vi "Accelerometer.vi"(1 "Mode":enum8{"Start", "Run", "Finish"}(ring)) -> (0 "Distances":cluster{"X":dbl, "Y":dbl, "Z":dbl})   [LabVIEW 2014]
uses:
  <vilib>/Rock Robotics/WPI/Accelerometer/InternalAccelerometer/WPI_AccelerometerInternalOpen.vi
  <vilib>/Analysis/NI_AALPro.lvlib
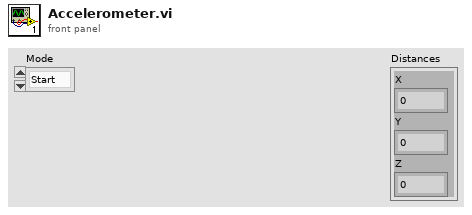
[diagram p1: front panel]
types:
  T1 = typedef "WPI_AccelerometerDevRef.ctl" = cluster{"DevStatus":errorcluster, "Controller":T2, "Scaling":T3, "Analog Channels":T4, "I2C Bus":T6, "SPI Bus":T7, "Accel Range":T8, "ADXL345 Axes":T9, "Handle":i32, "Device Address":u8, "Accel Type":enum16{"Analog", "ADXL345 I2C", "ADXL345 SPI", "Internal"}}
  T2 = typedef "FPGA_TypedefAnalogModule.ctl" = enum16{"Controller 1"}
  T3 = typedef "WPI_AccelerometerScaling.ctl" = cluster{"Gain (VoltsPerG)":dbl, "Center Voltage":dbl}
  T4 = typedef "WPI_AccelerometerAnalogChannels.ctl" = cluster{"X-Axis":T5, "Y-Axis":T5, "Z-Axis":T5}
  T5 = typedef "FPGA_AIChannel.ctl" = enum8{"AI 0", "AI 1", "AI 2", "AI 3", "AI MXP 0", "AI MXP 1", "AI MXP 2", "AI MXP 3", "Invalid"}
  T6 = typedef "i2c_bus.ctl" = enum16{"I2C On-Board", "I2C MXP", "Invalid"}
  T7 = typedef "spi_bus.ctl" = enum16{"SPI On-Board, CS0", "SPI On-Board, CS1", "SPI On-Board, CS2", "SPI On-Board, CS3", "SPI MXP", "Invalid"}
  T8 = typedef "ADXL345 Range.ctl" = u8
  T9 = typedef "WPI_AccelerometerADXL345 Axes.ctl" = cluster{"X-Axis":bool, "Y-Axis":bool, "Z-Axis":bool}
  T10 = cluster{"X-Axis":dbl, "Y-Axis":dbl, "Z-Axis":dbl}
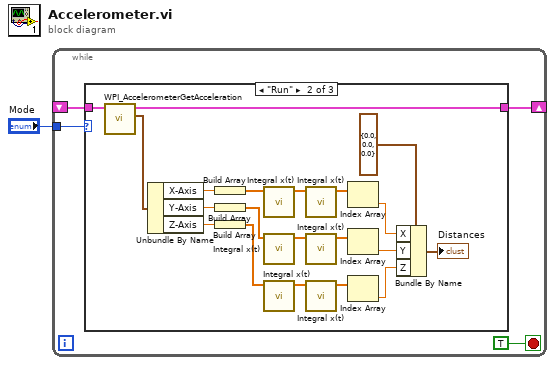
[diagram p0: block diagram]
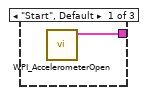
[diagram p2: hidden frame]
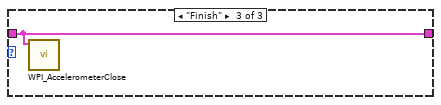
[diagram p3: hidden frame]
diagram:
  n1 = while {
    tunnel: "Mode" -> [w5]
    shift-right: [w4] -> _
    shift-left: _ -> [w3]
    stop <- TRUE stop-if-true
    n2 = case shown="\"Run\"" w5 {
      tunnel: [w6 w25 w27] -> w4
      tunnel: w3 -> [_ w26 w27]
      frame "Start", Default {
        n3 = call-poly <vilib>:"WPI_AccelerometerOpen.vi"() -> ("AccelerometerDevRef"=w6:T1)  [unwired: 10 in, 1 out]
      }
      frame "Run" {
        n4 = call <vilib>:"WPI_AccelerometerGetAcceleration.vi"("AccelerometerDevRef"=w26) -> ("Accelerations"=w24:T10, "AccelerometerDevRef"=w25:T1)  [unwired: 8 in, 1 out]
        n5 = Unbundle By Name(w24) -> ("X-Axis"=w23:dbl, "Y-Axis"=w20:dbl, "Z-Axis"=w17:dbl)
        n6 = Build Array(w23) -> (w22:dbl[])
        n7 = Build Array(w20) -> (w19:dbl[])
        n8 = Build Array(w17) -> (w16:dbl[])
        n9 = call <vilib>:"Integral x(t).vi"("X"=w22) -> ("Integral X"=w21:dbl[])  [unwired: 9 in, 1 out]
        n10 = call <vilib>:"Integral x(t).vi"("X"=w19) -> ("Integral X"=w18:dbl[])  [unwired: 9 in, 1 out]
        n11 = call <vilib>:"Integral x(t).vi"("X"=w16) -> ("Integral X"=w15:dbl[])  [unwired: 9 in, 1 out]
        n12 = call <vilib>:"Integral x(t).vi"("X"=w21) -> ("Integral X"=w13:dbl[])  [unwired: 9 in, 1 out]
        n13 = call <vilib>:"Integral x(t).vi"("X"=w18) -> ("Integral X"=w11:dbl[])  [unwired: 9 in, 1 out]
        n14 = call <vilib>:"Integral x(t).vi"("X"=w15) -> ("Integral X"=w9:dbl[])  [unwired: 9 in, 1 out]
        n15 = Index Array(array=w13) -> (element=w12:dbl)  [unwired: 1 in]
        n16 = Index Array(array=w11) -> (element=w10:dbl)  [unwired: 1 in]
        n17 = Index Array(array=w9) -> (element=w8:dbl)  [unwired: 1 in]
        n18 = Bundle By Name(cluster=cluster{"X":dbl, "Y":dbl, "Z":dbl} {"X"=0.0, "Y"=0.0, "Z"=0.0} ("Distances"), "X"=w12, "Y"=w10, "Z"=w8) -> (→"Distances":cluster{"X":dbl, "Y":dbl, "Z":dbl})
      }
      frame "Finish" {
        n19 = call <vilib>:"WPI_AccelerometerClose.vi"("AccelerometerDevRef"=w27) -> ()  [unwired: 10 in, 1 out]
      }
    }
  }
